vi "Grader Test Helper.vi"() -> ()   [LabVIEW 2013]
uses:
  VIChallenge.lvlib
panel:
  out "Error Out":errorcluster
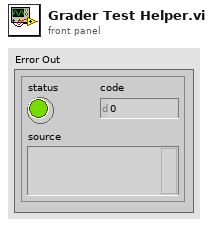
[diagram p1: front panel]
types:
  T1 = typedef "VIChallenge.lvlib/VIChallenge Config.ctl" = cluster{"AWS Credentials":T2, "AWS Account Number":string, "SQS Jobs":refnum<class "AWS_SQS.lvclass">, "SQS Status":refnum<class "AWS_SQS.lvclass">, "Source Dir":path, "Working Dir":path, "Output Dir":path, "Archive Dir":path, "job":T3, "Database Ref":T4, "Challenge Dir":path, "Challenges":T5[]}
  T2 = typedef "AWS_Core.lvlib/AWS_AWS Credentials.ctl" = cluster{"AWSAccessKeyId":string, "Secret Key":string}
  T3 = typedef "VIChallenge.lvlib/JSON_job.ctl" = cluster{"job_id":string, "challenge_id":string, "user_id":string, "s3_source_bucket":string, "s3_source_directory":string, "s3_source_filename":string, "status_queue_name":string, "username":string}
  T4 = typedef "NI_Database_API.lvlib/Conn ObjectReference.ctl" = refnum<k1>
  T5 = typedef "VIChallenge.lvlib/Challenge.ctl" = cluster{"General":cluster{"Challenge Id":i32, "Template Name":string}, "Unit Test Framework":cluster{"Enabled Unit Test Templates":path[]}, "VI Analyzer":cluster{"Enabled VI Analyzer Tests":path[]}, "Custom Tests":cluster{"Enabled Custom Tests":path[]}}
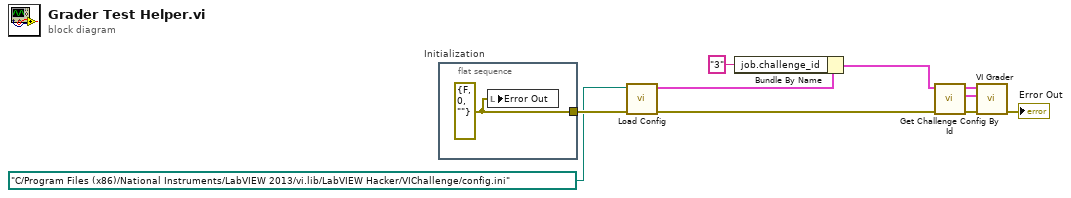
[diagram p0: block diagram]
diagram:
  n1 = flat-sequence "Initialization" {
    tunnel: [w11] -> w10
    frame #0 {
      w11 = errorcluster {"status"=FALSE, "code"=0, "source"=""} ("Error Out")
      n2 = local write "Error Out"(w11) -> ()
    }
  }
  n3 = call "Load Config.vi"("Error In"=w10, "Config File Path Override"=path "C:/Program Files (x86)/National Instruments/LabVIEW 2013/vi.lib/LabVIEW Hacker/VIChallenge/config.ini") -> ("Error Out"=w6:errorcluster, "VIChallenge Config"=w2:T1)  [unwired: 8 in]
  n4 = Bundle By Name(cluster=w2, "job.challenge_id"="3") -> (w3:T1)
  n5 = call "Get Challenge Config By Id.vi"("Error In"=w6, "VIChallenge Config"=w3) -> ("Error Out"=w7:errorcluster, "Challenge Config"=w9:T5, "VIChallenge Config"=w8:T1)  [unwired: 7 in]
  n6 = call "VI Grader.vi"("Error In"=w7, "Challenge Config"=w9, "VIChallenge Config"=w8) -> ("Error Out"=→"Error Out":errorcluster)  [unwired: 6 in, 2 out]
